vi "ME_acquire_6.vi"() -> ()   [LabVIEW 2015]
doc: "Use this template to build a producer/consumer design pattern. Use this template when you need to execute a process, such as data analysis, when a data source, such as a triggered acquisition, produces data at an uneven rate and you need to execute the process when the data becomes available."
uses:
  Mode.ctl
  oxford_driver/Oxford Drivers/BUSGEN.LLB/OxfordAddress.ctl
  <vilib>/Analysis/baseanly.llb/Mean (DBL).vi
  <vilib>/Utility/file.llb/Write Delimited Spreadsheet (DBL).vi
  <vilib>/express/express arith-compare/Formula/XNode/ExpressFormulaBlockNode.xnode
  <vilib>/gmath/NI_Gmath.lvlib
  <vilib>/Analysis/NI_AALBase.lvlib
panel:
  out "I(B) /Averaged/ 2":cluster{"B array":dbl[], dbl[]}[](graph)
  out "Averaged I(B)":dbl[][](array[numeric])
  out "P(uC/mm^2)":dbl[](array[numeric])
  in  "Sweep Field":bool
  out "P(B)":cluster{"yi":dbl[], dbl[]}(graph)
  out "Offset array":dbl[](array[numeric])
  in  "stop 2":bool
  in  "dB":dbl=0.005
  in  "Dwell Time (ms)":u32=1
  out "appended array":dbl[][](array[numeric])
  in  "Magnet":bool
  out "Actual B Field (T)":dbl
  out "Actual Temperature (K)":dbl
  out "Actual Current (pA)":dbl
  in  "Tab Control":T1(tab)
  out "P(T)":cluster{"yi":dbl[], dbl[]}(graph)
  out "I(T)":cluster{dbl[], dbl[]}(graph)
  in  "Set temperature (K)":dbl=4.5
  in  "Temp Ramping Rate (K/min)":dbl=10.0
  in  "Heater Range":enum16{"Off", "Low", "Medium", "High"}(ring)
  in  "Heater On/Off":bool
  out "I(B) /Averaged/":cluster{"B array":dbl[], dbl[]}[](graph)
  out "I(B) 3":cluster{dbl[], dbl[]}[](graph)
  in  "Go to Set":bool
  in  "Set Field (T)":dbl=0.3
  in  "Field To Zero":bool
  in  "Sweep Rate (T/min)":dbl=2.0 format="%.6f"
  in  "Min Field (T)":dbl
  in  "Max Field (T)":dbl
  out "Up/Down":bool
  in  "Measure Noise":bool
  in  "Cycles":i32
  in  "maximum value":dbl=10.0 format="%0.2f"
  in  "minimum value":dbl=-10.0 format="%0.2f"
  in  "physical channels":tag="Dev1/ai1"
  out "PSD (pA/Hz^1/2) Peaks Removed":cluster{"f0":dbl, "df":dbl, "magnitude":dbl[]}(graph)
  out "PSD (pA/Hz^1/2)":cluster{"f0":dbl, "df":dbl, "magnitude":dbl[]}(graph)
  out "Current (pA) Filtered":waveform(dbl)(graph)
  out "Current (pA)":dbl[](graph)
  in  "Samples per channel":i32=1000
  in  "Rate":dbl=1000.0 format="%0.2f"
  in  "Cut-Off Frequency":dbl=100.0 caption="Lower Cut-Off"
  in  "Filter On":bool
  out "Dc offset":dbl
  in  "Calibrate":bool
  in  "IV converter":refnum<visa-resource-name>="GPIB0::20::INSTR"
  in  "Magnetic Field":refnum<visa-resource-name>="GPIB0::21::INSTR"
  out "Time Lag":dbl=0.0500025749206543
  in  "Lake Shore":refnum<visa-resource-name>="GPIB0::11::INSTR"
  in  "Temp Refresh (s)":dbl=1.0
  in  "Sampling rate (Hz)":dbl=10.0
  in  "Gain (V/A)":dbl=1000000000.0
  in  "Sample area (mm^2)":dbl=3.9
  out "B_V":cluster{dbl[], "Best Linear Fit":dbl[]}[](graph)=[{[-0.00854253601, 0.00626134724, 0.0219834428, 0.0379117736, 0.0535871506, 0.0694316728, 0.0851615152, 0.100816481, 0.116478038, 0.132148461, 0.147876163, 0.16341701, 0.178976744, 0.194563632, 0.210251739, 0.225738944, 0.241298253, 0.256806034, 0.272344374, 0.287933477, 0.303494709, 0.318997125, 0.334591297, 0.350146681, 0.365618053, 0.380940961, 0.39666457, 0.412213675, 0.427724671, 0.443221444, 0.458760641, 0.474360042, 0.489915118, 0.505330598, 0.520967119, 0.536347531, 0.551813711, 0.567441155, 0.582995861, 0.598507522, 0.614041988, 0.629563151, 0.645106262, 0.660611914, 0.676136149, 0.691553948, 0.7071244, 0.72262999, 0.738171137, 0.753700392, 0.76919513, 0.784778028, 0.800215944, 0.8156961, 0.831325434, 0.846852183, 0.862326812, 0.877819169, 0.893312568, 0.90888536, 0.924354789], "Best Linear Fit"=[0.0, 0.005, 0.01, 0.015, 0.02, 0.025, 0.03, 0.035, 0.04, 0.045, 0.05, 0.055, 0.06, 0.065, 0.07, 0.075, 0.08, 0.085, 0.09, 0.095, 0.1, 0.105, 0.11, 0.115, 0.12, 0.125, 0.13, 0.135, 0.14, 0.145, 0.15, 0.155, 0.16, 0.165, 0.17, 0.175, 0.18, 0.185, 0.19, 0.195, 0.2, 0.205, 0.21, 0.215, 0.22, 0.225, 0.23, 0.235, 0.24, 0.245, 0.25, 0.255, 0.26, 0.265, 0.27, 0.275, 0.28, 0.285, 0.29, 0.295, 0.3]}, {[-0.00854253601, 0.00626134724, 0.0219834428, 0.0379117736, 0.0535871506, 0.0694316728, 0.0851615152, 0.100816481, 0.116478038, 0.132148461, 0.147876163, 0.16341701, 0.178976744, 0.194563632, 0.210251739, 0.225738944, 0.241298253, 0.256806034, 0.272344374, 0.287933477, 0.303494709, 0.318997125, 0.334591297, 0.350146681, 0.365618053, 0.380940961, 0.39666457, 0.412213675, 0.427724671, 0.443221444, 0.458760641, 0.474360042, 0.489915118, 0.505330598, 0.520967119, 0.536347531, 0.551813711, 0.567441155, 0.582995861, 0.598507522, 0.614041988, 0.629563151, 0.645106262, 0.660611914, 0.676136149, 0.691553948, 0.7071244, 0.72262999, 0.738171137, 0.753700392, 0.76919513, 0.784778028, 0.800215944, 0.8156961, 0.831325434, 0.846852183, 0.862326812, 0.877819169, 0.893312568, 0.90888536, 0.924354789], "Best Linear Fit"=[-0.00022554388023060128, 0.004536267537808887, 0.009593430775915074, 0.014716931562355689, 0.01975906732634002, 0.024855610270593523, 0.029915265354287977, 0.03495083565949541, 0.03998852608757118, 0.045029068349812316, 0.05008803495326229, 0.055086897848955874, 0.060091835929837946, 0.06510550835596321, 0.07015173884687344, 0.07513334727738563, 0.08013814865293042, 0.08512637555172443, 0.0901244320467579, 0.09513881694893507, 0.10014423687592358, 0.10513073807087174, 0.11014675346564809, 0.1151502923271957, 0.12012680792099008, 0.1250555686413888, 0.1301132186920259, 0.13511473785283767, 0.14010399888730068, 0.14508868495702945, 0.1500870171143548, 0.15510471446726903, 0.16010815425765457, 0.16506669165212906, 0.17009632901003072, 0.1750435864450521, 0.18001843198211442, 0.1850451496356715, 0.19004847041199868, 0.1950379453501071, 0.20003475573578386, 0.20502728708357412, 0.21002687821664084, 0.21501442030211, 0.220007939788244, 0.2249672231113706, 0.22997560874002893, 0.23496313088260184, 0.23996209027618054, 0.24495722449359253, 0.24994125598600042, 0.2549536449902534, 0.25991939913989753, 0.2648987401917687, 0.26992606578200207, 0.2749203939204135, 0.2798979571595809, 0.2848812227804405, 0.2898648235706211, 0.2948739618827834, 0.2998498524919418]}]
  out "V_I":cluster{dbl[], "Best Linear Fit":dbl[]}[](graph)=[{[0.0, 0.035, 0.069, 0.104, 0.138, 0.173, 0.208, 0.242, 0.277, 0.311, 0.346, 0.38, 0.415, 0.45, 0.484, 0.519, 0.553, 0.588, 0.623, 0.657, 0.692, 0.726, 0.761, 0.796, 0.83, 0.865, 0.899, 0.934, 0.969, 1.003, 1.038, 1.072, 1.107, 1.141, 1.176, 1.211, 1.245, 1.28, 1.314, 1.349, 1.384, 1.418, 1.453, 1.487, 1.522, 1.557, 1.591, 1.626, 1.66, 1.695, 1.73, 1.764, 1.799, 1.833, 1.868, 1.902, 1.937, 1.972, 2.006, 2.041, 2.075], "Best Linear Fit"=[-0.00854253601, 0.00626134724, 0.0219834428, 0.0379117736, 0.0535871506, 0.0694316728, 0.0851615152, 0.100816481, 0.116478038, 0.132148461, 0.147876163, 0.16341701, 0.178976744, 0.194563632, 0.210251739, 0.225738944, 0.241298253, 0.256806034, 0.272344374, 0.287933477, 0.303494709, 0.318997125, 0.334591297, 0.350146681, 0.365618053, 0.380940961, 0.39666457, 0.412213675, 0.427724671, 0.443221444, 0.458760641, 0.474360042, 0.489915118, 0.505330598, 0.520967119, 0.536347531, 0.551813711, 0.567441155, 0.582995861, 0.598507522, 0.614041988, 0.629563151, 0.645106262, 0.660611914, 0.676136149, 0.691553948, 0.7071244, 0.72262999, 0.738171137, 0.753700392, 0.76919513, 0.784778028, 0.800215944, 0.8156961, 0.831325434, 0.846852183, 0.862326812, 0.877819169, 0.893312568, 0.90888536, 0.924354789]}, {[0.0, 0.035, 0.069, 0.104, 0.138, 0.173, 0.208, 0.242, 0.277, 0.311, 0.346, 0.38, 0.415, 0.45, 0.484, 0.519, 0.553, 0.588, 0.623, 0.657, 0.692, 0.726, 0.761, 0.796, 0.83, 0.865, 0.899, 0.934, 0.969, 1.003, 1.038, 1.072, 1.107, 1.141, 1.176, 1.211, 1.245, 1.28, 1.314, 1.349, 1.384, 1.418, 1.453, 1.487, 1.522, 1.557, 1.591, 1.626, 1.66, 1.695, 1.73, 1.764, 1.799, 1.833, 1.868, 1.902, 1.937, 1.972, 2.006, 2.041, 2.075], "Best Linear Fit"=[-0.007846580254753975, 0.007882153481927697, 0.02316149482613275, 0.03889022856281441, 0.054169569907019474, 0.06989830364370113, 0.08562703738038281, 0.10090637872458785, 0.11663511246126955, 0.1319144538054746, 0.14764318754215625, 0.1629225288863613, 0.17865126262304296, 0.19437999635972467, 0.2096593377039297, 0.22538807144061138, 0.24066741278481643, 0.25639614652149806, 0.27212488025817977, 0.2874042216023848, 0.3031329553390665, 0.31841229668327153, 0.3341410304199532, 0.3498697641566349, 0.3651491055008399, 0.3808778392375216, 0.39615718058172666, 0.4118859143184083, 0.42761464805509, 0.442893989399295, 0.45862272313597674, 0.4739020644801818, 0.48963079821686345, 0.5049101395610684, 0.5206388732977502, 0.5363676070344319, 0.5516469483786369, 0.5673756821153185, 0.5826550234595236, 0.5983837571962053, 0.6141124909328869, 0.629391832277092, 0.6451205660137737, 0.6603999073579787, 0.6761286410946604, 0.691857374831342, 0.7071367161755471, 0.7228654499122288, 0.7381447912564338, 0.7538735249931156, 0.7696022587297972, 0.7848816000740022, 0.8006103338106839, 0.815889675154889, 0.8316184088915707, 0.8468977502357756, 0.8626264839724573, 0.878355217709139, 0.893634559053344, 0.9093632927900257, 0.9246426341342309]}]
  out "B0 (T)":dbl=0.0025222449819540214
  out "B/V (T/V)":dbl=0.321659617116981
  out "I0 (A)":dbl=-0.007846580254753975
  out "V/I (Ohm)":dbl=0.44939239247661916
  in  "Offset?":bool
  in  "Temp/Magnetic Field":bool
  out "Save":dbl[][](array[numeric])
  out "output array":dbl[][](array[numeric])
  out "index":i8
  out "Read?":bool
  out "Magnetic Field (T)":dbl[](array[numeric])
  out "Reset":bool
  out "Measured Current (pA)":dbl[](array[numeric])
  out "Elapsed Time (s)":dbl[](array[numeric])
  out "Start time":timestamp
  in  "Enum":T2=enum."Process"
  out "B array":dbl[](array[numeric])
  in  "dB (T)":dbl=0.0001
  in  "Counter":i8
  out "L magnet (H)":dbl
  out "R magnet (mOhm)":dbl
  out "Actual Current (R0)":dbl
  out "Actual Field (T)":dbl
  out "Temperature array":dbl[](array[numeric])
  in  "New Measurement File":bool
  out "Measurement File":path
  out "refnum out":refnum<file>
  in  "Measuring":bool
  in  "Measure (Start/Pause)":bool
  in  "stop":bool
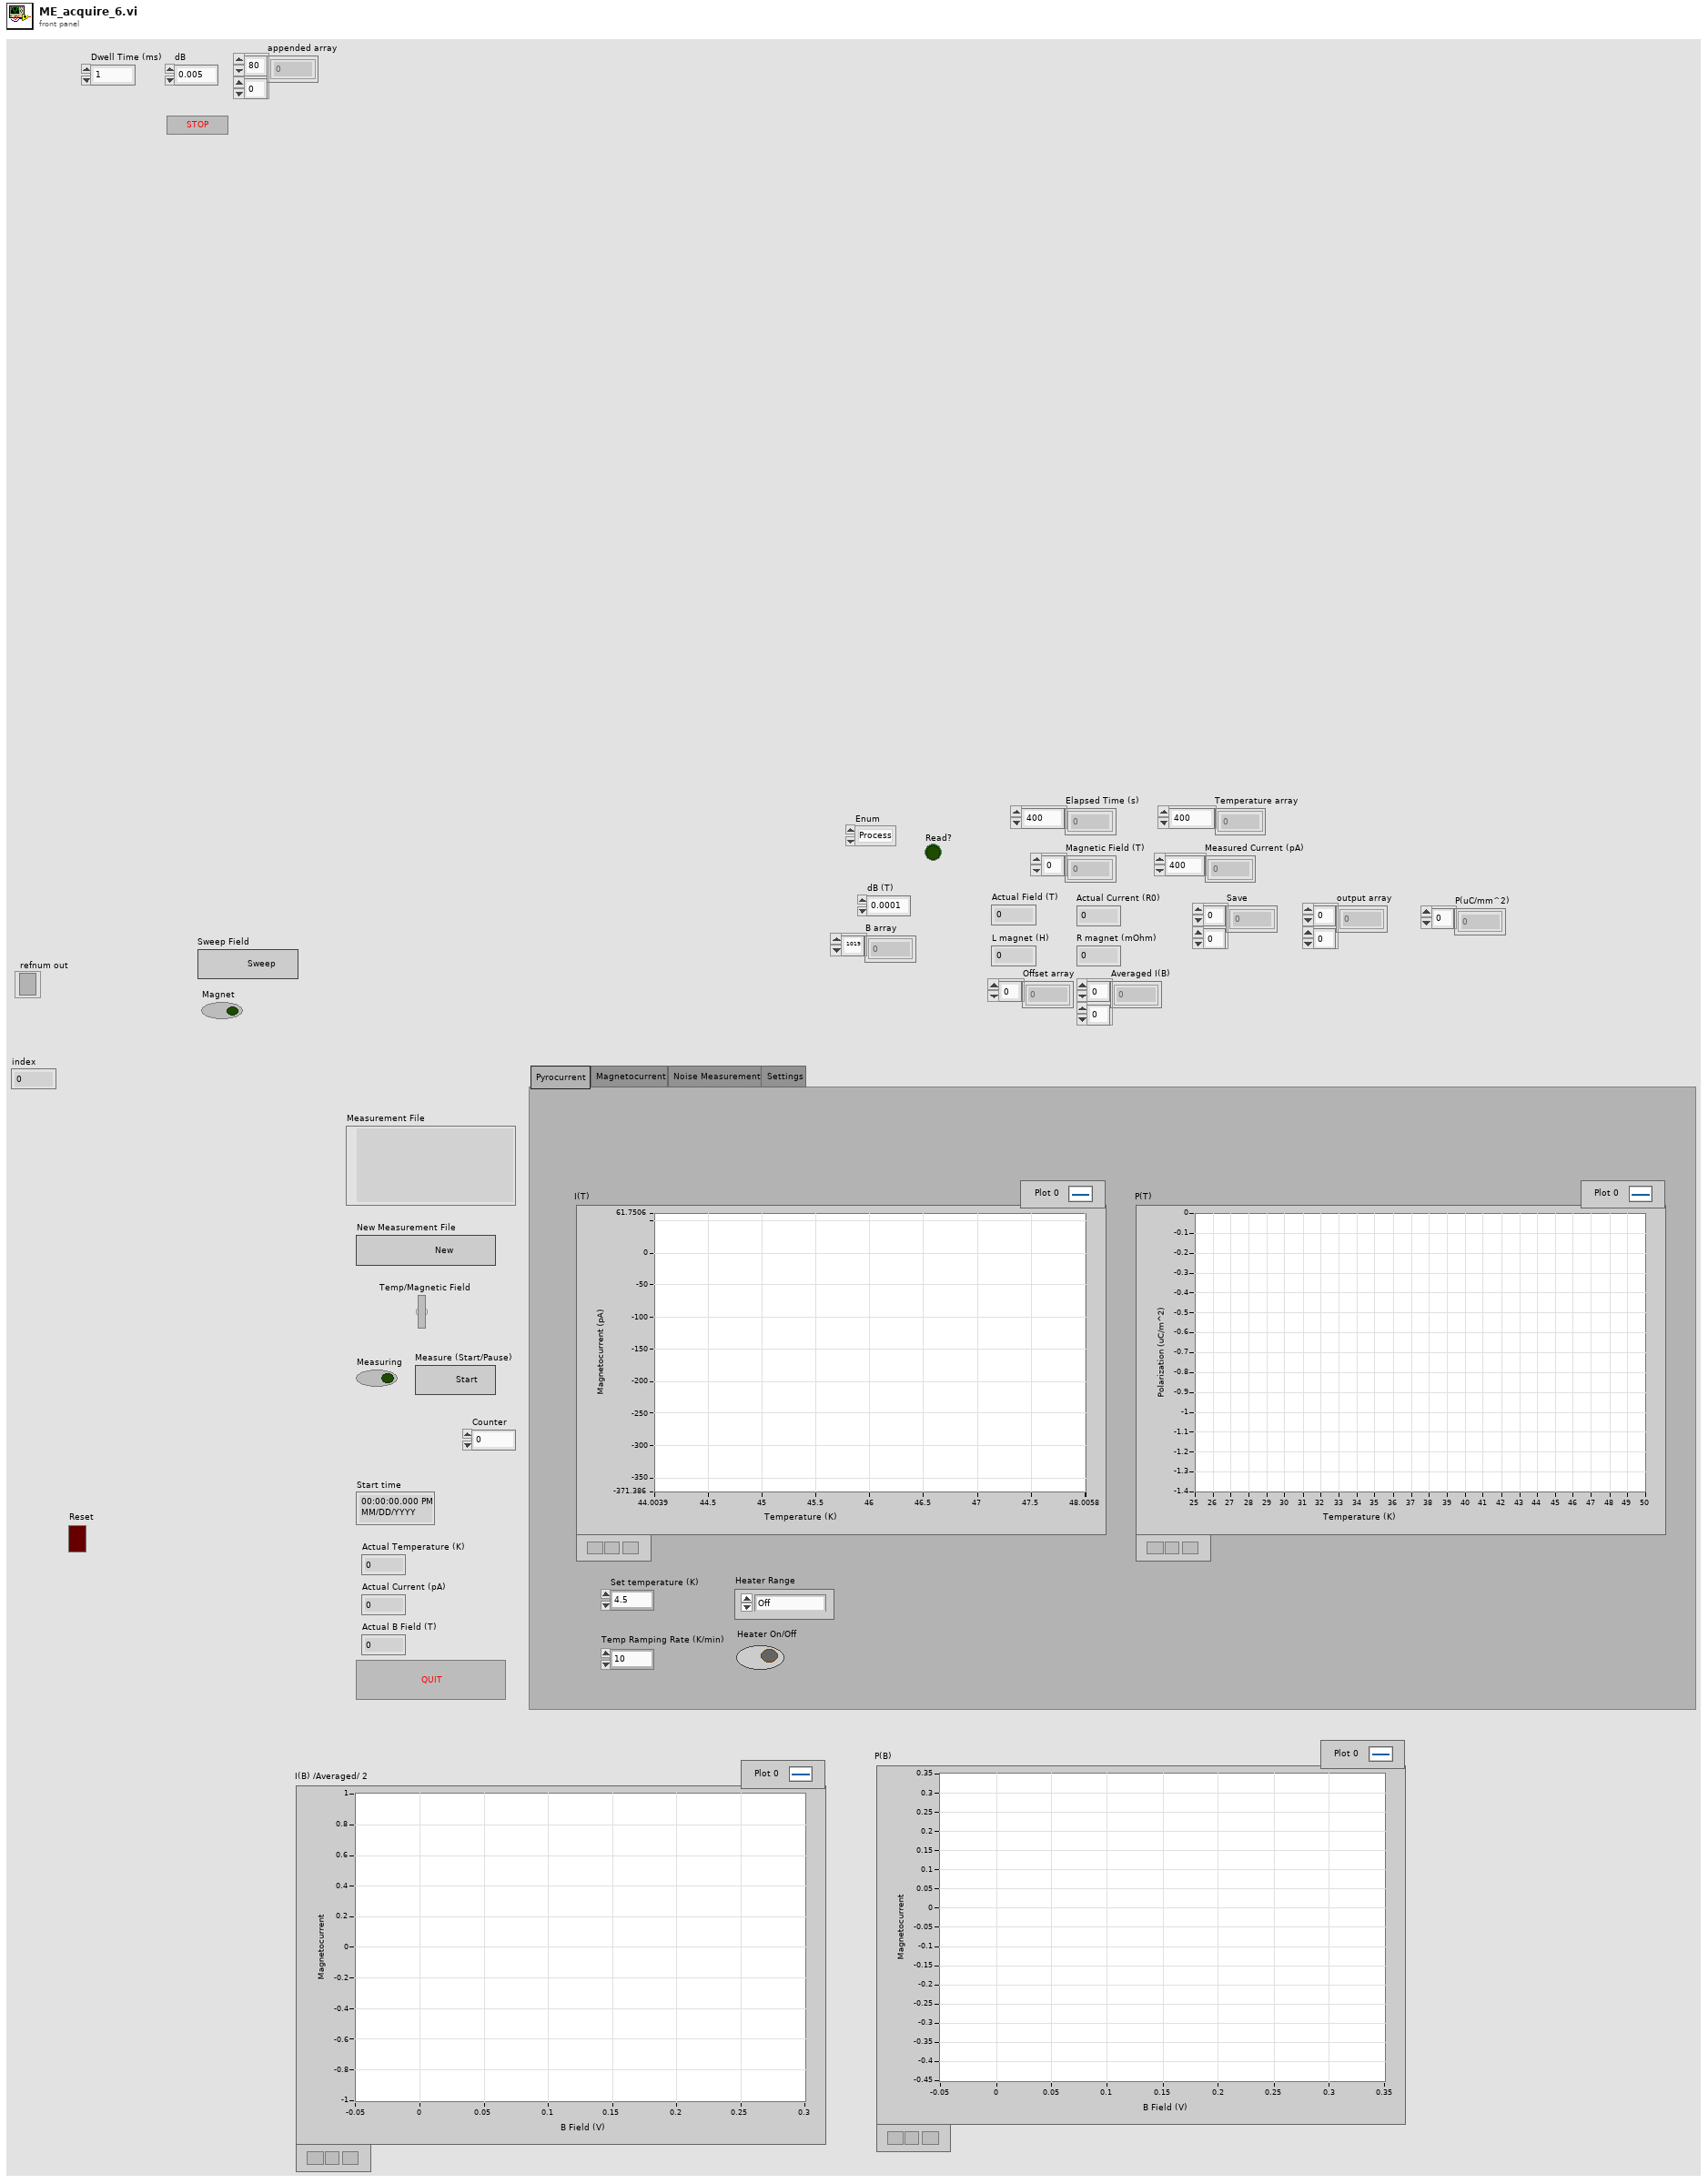
[diagram p1: front panel]
types:
  T1 = enum32{"Pyrocurrent", "Magnetocurrent", "Noise Measurement", "Settings"}
  T2 = typedef "Mode.ctl" = enum16{"Offset", "Process", "Sweep", "Plot", "Save", "Return"}
  T3 = enum16{"open", "replace", "create", "open or create", "replace or create", "replace or create with confirmation"}
  T4 = typedef "OxfordAddress.ctl" = cluster{"Com Port":i32, "ISOBUS Address":i32, "GPIB Address":i16, "Communication":enum16{"RS232", "ISOBUS", "GPIB", "Gateway"}}
  T5 = cluster{"seconds since 1Jan1904":timestamp, "read buffer":string, "read buffer":string}
  T6 = cluster{"B array":dbl[], "Averaged I(B) out":dbl[]}
  T7 = cluster{"B array":dbl[], "Averaged I(B) out":dbl[]}[]
  T8 = cluster{"I array out (A)":dbl[], "V array out (V)":dbl[]}
  T9 = cluster{"I array out (A)":dbl[], "Best Linear Fit":dbl[]}
  T10 = cluster{"V array out (V)":dbl[], "B array Out":dbl[]}
  T11 = cluster{"V array out (V)":dbl[], "Best Linear Fit 2":dbl[]}
  T12 = cluster{"I array out (A)":dbl[], "Best Linear Fit":dbl[]}[]
  T13 = cluster{"V array out (V)":dbl[], "Best Linear Fit 2":dbl[]}[]
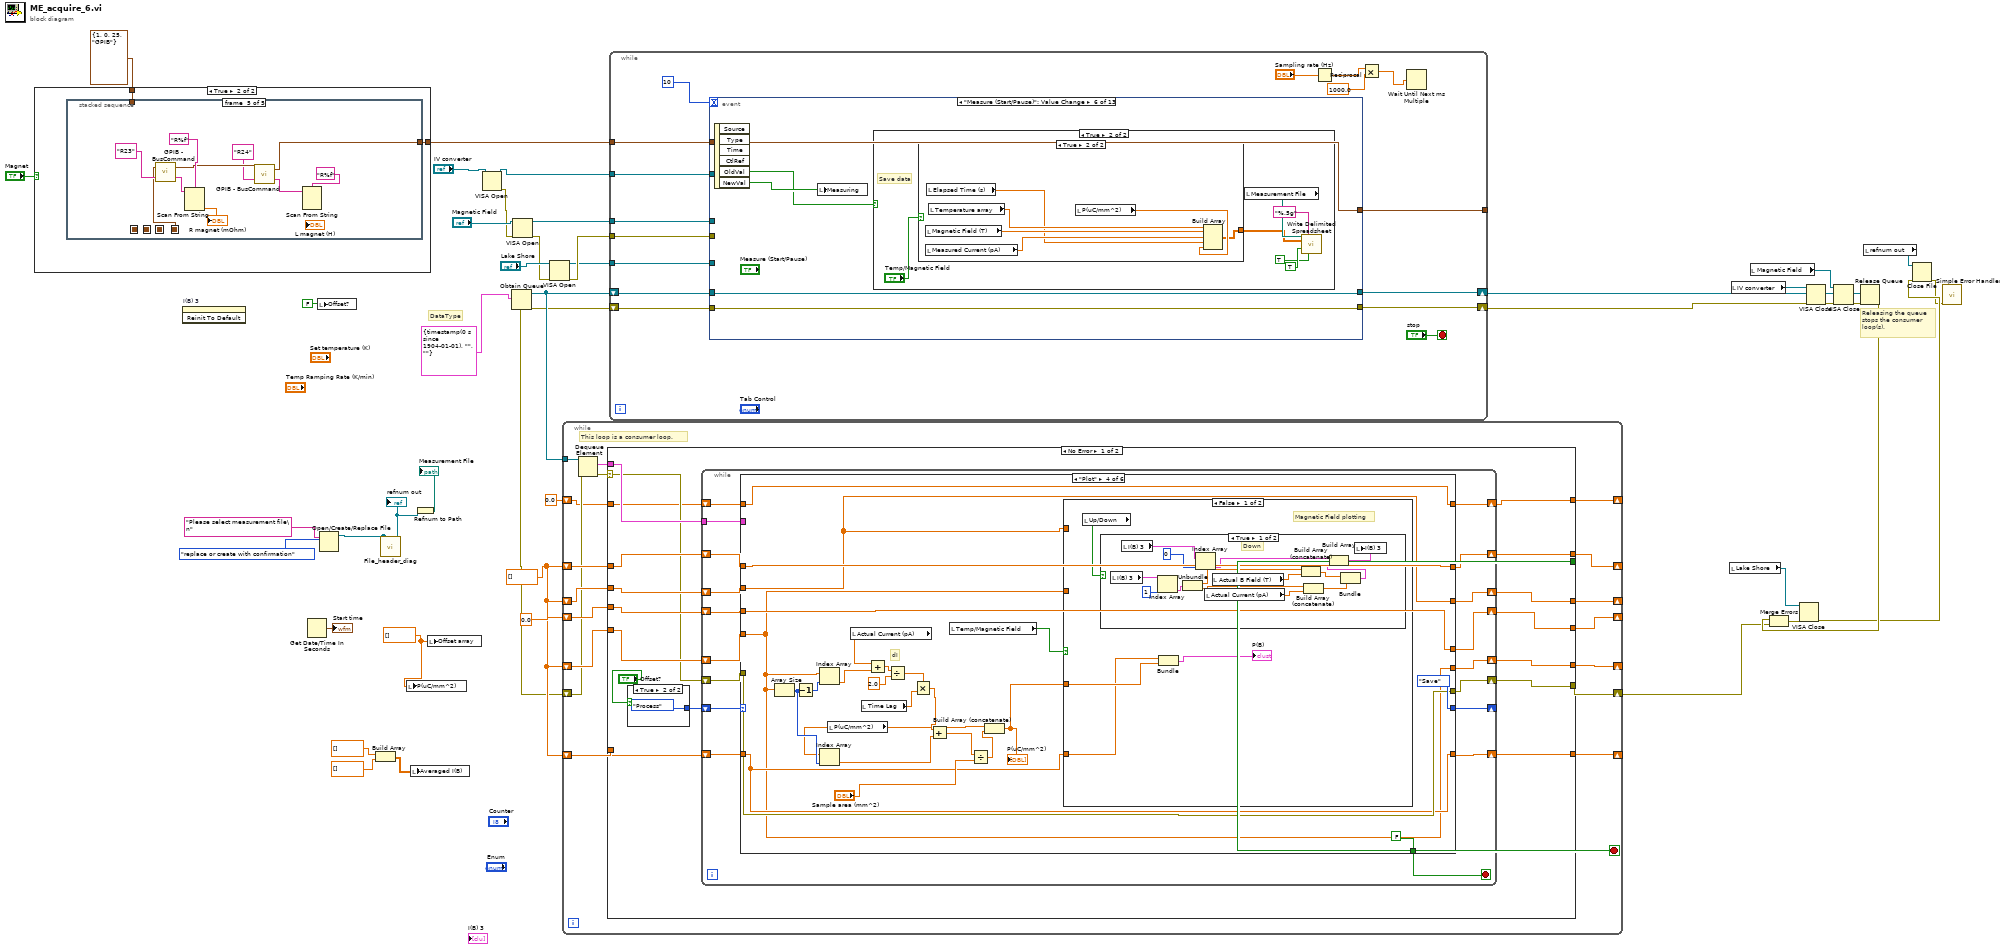
[diagram p0: block diagram]
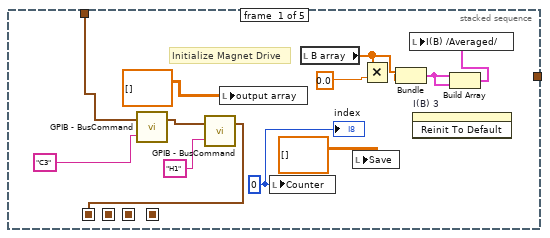
[diagram p3: hidden frame]
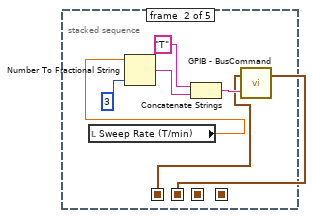
[diagram p4: hidden frame]
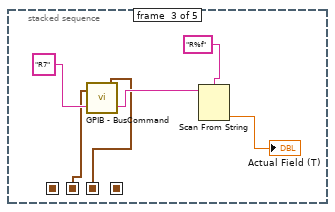
[diagram p5: hidden frame]
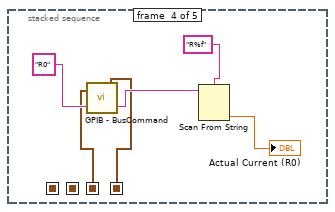
[diagram p6: hidden frame]
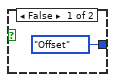
[diagram p7: hidden frame]
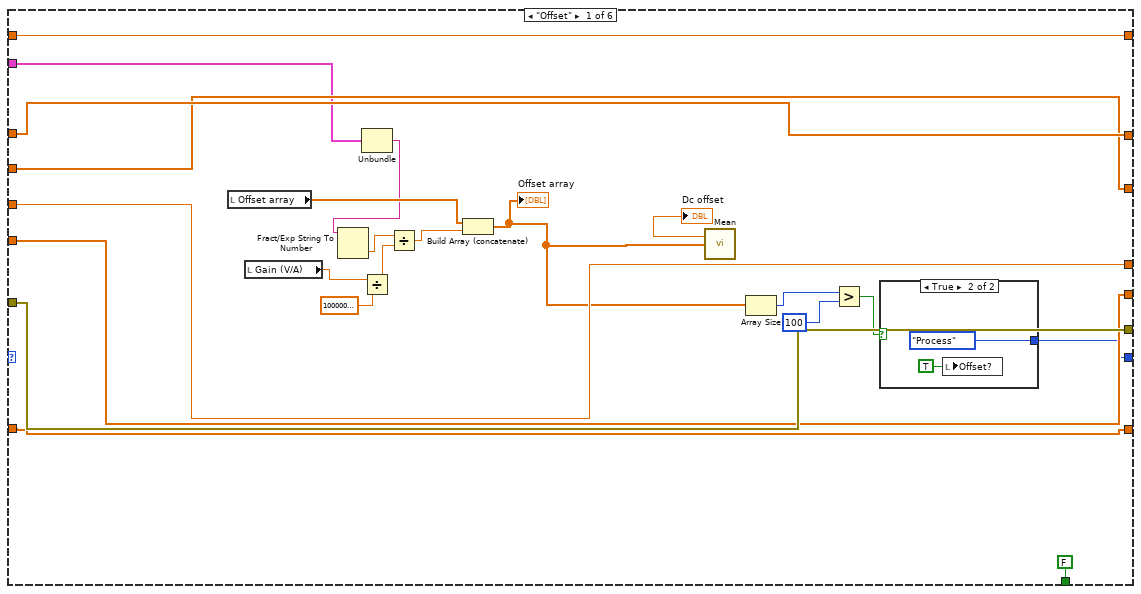
[diagram p8: hidden frame]
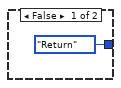
[diagram p9: hidden frame]
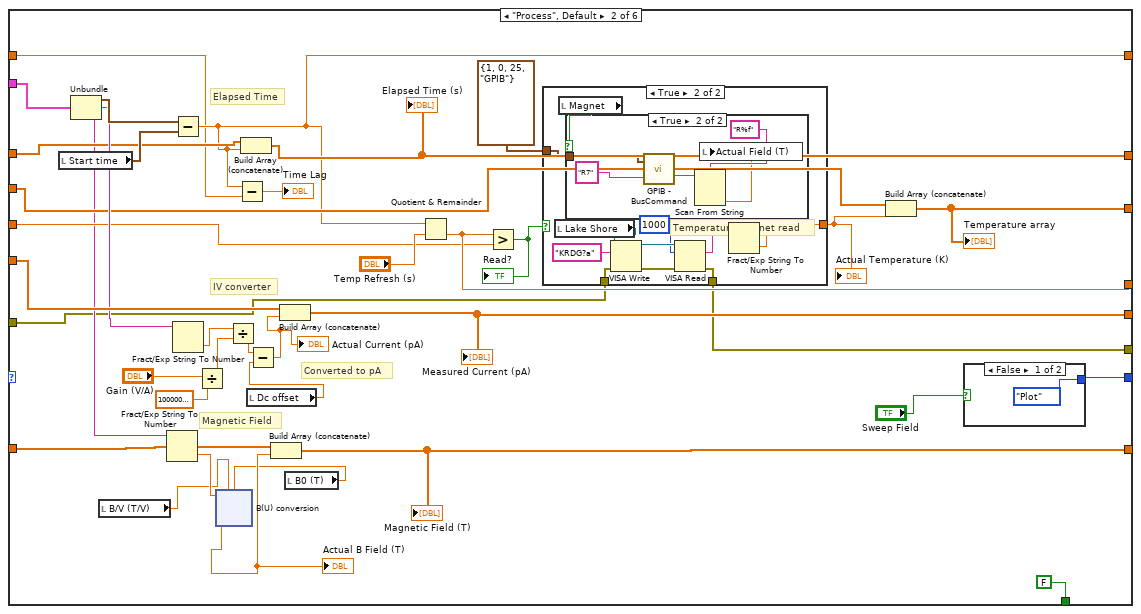
[diagram p10: hidden frame]
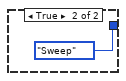
[diagram p11: hidden frame]
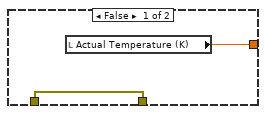
[diagram p12: hidden frame]
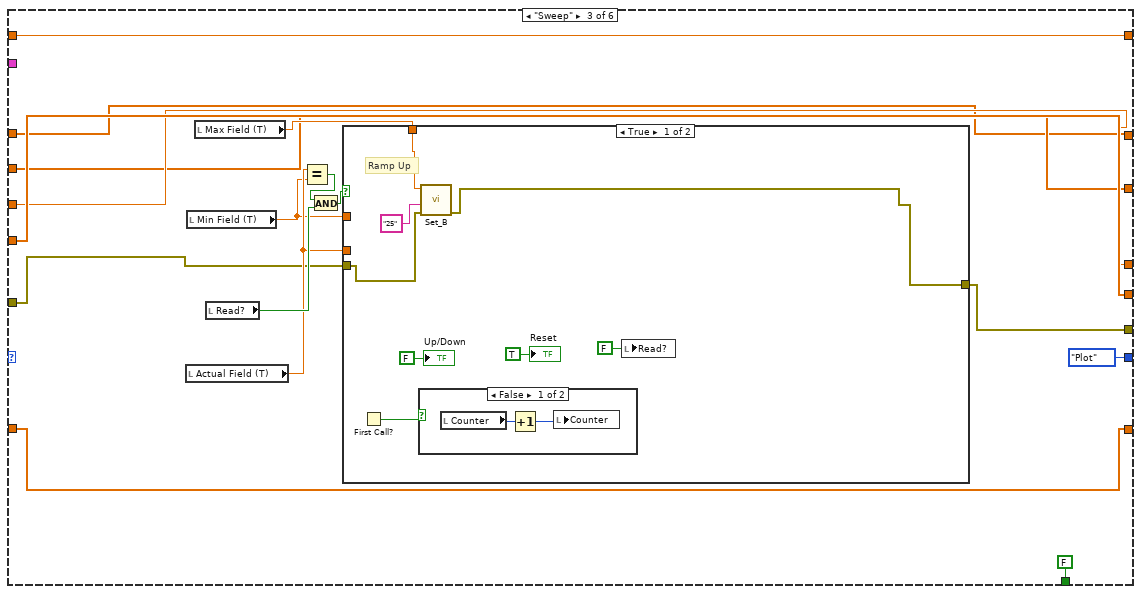
[diagram p14: hidden frame]
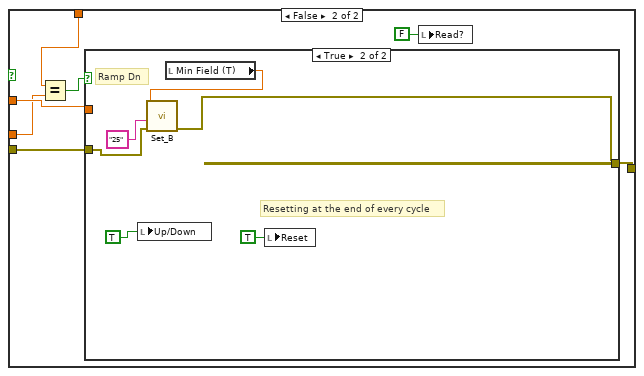
[diagram p16: hidden frame]
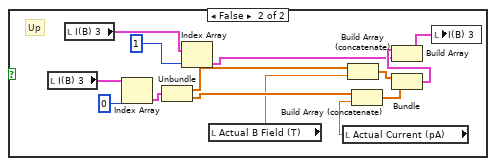
[diagram p18: hidden frame]
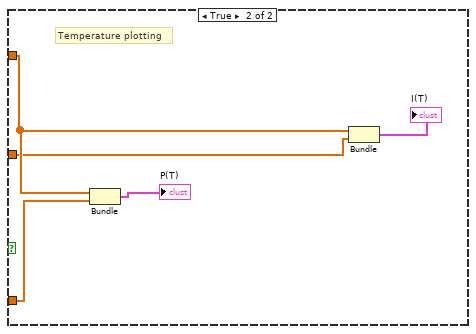
[diagram p19: hidden frame]
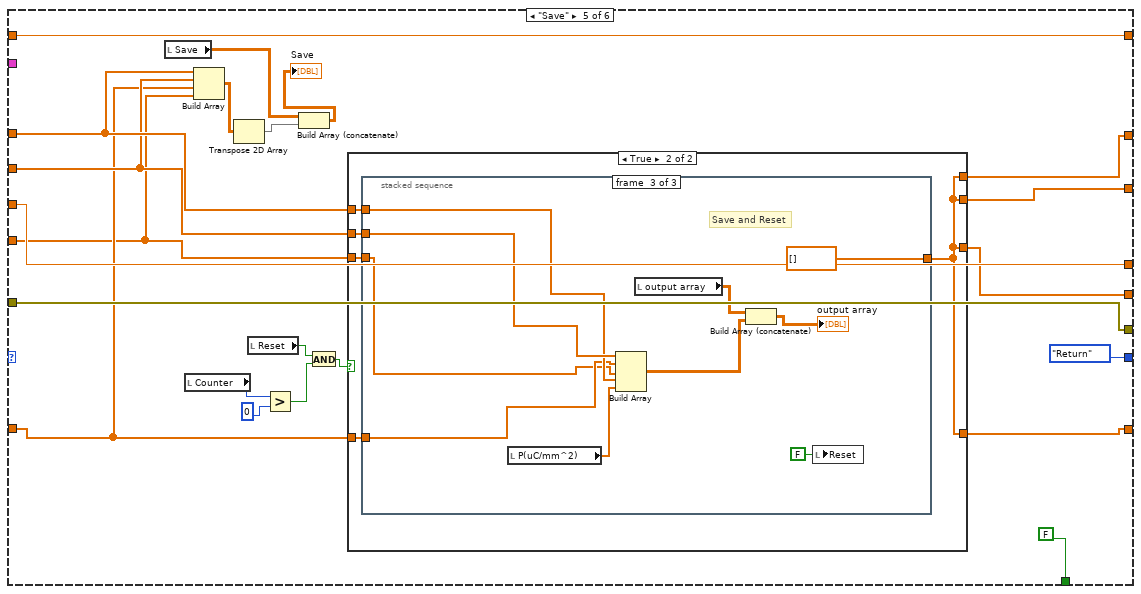
[diagram p20: hidden frame]
diagram:
  w4 = dbl[] []
  w11 = dbl[] []
  # "DataType"
  # "Releasing the queue stops the consumer loop(s)."
  n1 = case shown="True" "Magnet" {
    tunnel: T4 {"Com Port"=1, "ISOBUS Address"=0, "GPIB Address"=25, "Communication"=enum."GPIB"} ("Address") -> [w42 w44]
    tunnel: [w42 w43] -> w20
    frame False {
    }
    frame True {
      n2 = stacked-sequence {
        seq-local: [w54 _ _ _ _] -> [_ w59 _ _ _]
        seq-local: [_ w58 _ _ _] -> [_ _ w66 _ _]
        seq-local: [_ _ w65 _ _] -> [_ _ _ w72 _]
        seq-local: [_ _ _ w71 _] -> [_ _ _ _ w82]
        tunnel: w44 -> [w56 _ _ _ _]
        tunnel: [_ _ _ _ w80] -> w43
        frame #0 {
          w52 = i8 0 ("Counter")
          # "Initialize Magnet Drive"
          n3 = call "GPIB - BusCommand.vi"("Command"="C3", "Address"=w56) -> ("Address(thru)"=w55:T4)  [unwired: 1 out]
          n4 = call "GPIB - BusCommand.vi"("Command"="H1", "Address"=w55) -> ("Address(thru)"=w54:T4)  [unwired: 1 out]
          n5 = local write "output array"(dbl[][] []) -> ()
          n6 = local write "Counter"(w52) -> ()
          n7 = local read "B array"() -> (w50:dbl[])
          n8 = local write "Save"(dbl[][] [] ("Save")) -> ()
          n9 = Multiply(x=w50, y=0.0) -> (x*y=w49:dbl[])
          n10 = Bundle("B array"=w50, w49) -> (w48:cluster{"B array":dbl[], dbl[]})  [unwired: 1 in]
          n11 = invoke on="I(B) 3" class="XYGraph (strict)" method="Reinit To Default"() -> ()  [unwired: 3 in, 3 out]
          n12 = Build Array(w48, w48) -> (w47:cluster{"B array":dbl[], dbl[]}[])
          n13 = local write "I(B) /Averaged/"(w47) -> ()
          "index" <- w52
        }
        frame #1 {
          n14 = local read "Sweep Rate (T/min)"() -> (w60:dbl)
          n15 = Number To Fractional String(number=w60, precision (6)=i16 3) -> (F-format string=w62:string)  [unwired: 2 in]
          n16 = Concatenate Strings("T" ("format string"), w62) -> (w61:string)
          n17 = call "GPIB - BusCommand.vi"("Command"=w61, "Address"=w59) -> ("Address(thru)"=w58:T4)  [unwired: 1 out]
        }
        frame #2 {
          n18 = call "GPIB - BusCommand.vi"("Command"="R7" ("format string"), "Address"=w66) -> ("Reply"=w70:string, "Address(thru)"=w65:T4)
          n19 = Scan From String(format string="R%f" ("remaining string"), input string=w70) -> (output 1=→"Actual Field (T)":dbl)  [unwired: 3 in, 3 out]
        }
        frame #3 {
          n20 = call "GPIB - BusCommand.vi"("Command"="R0" ("format string"), "Address"=w72) -> ("Reply"=w76:string, "Address(thru)"=w71:T4)
          n21 = Scan From String(format string="R%f" ("remaining string"), input string=w76) -> (output 1=→"Actual Current (R0)":dbl)  [unwired: 3 in, 3 out]
        }
        frame #4 {
          n22 = call "GPIB - BusCommand.vi"("Command"="R23" ("format string"), "Address"=w82) -> ("Reply"=w86:string, "Address(thru)"=w81:T4)
          n23 = Scan From String(format string="R%f" ("remaining string"), input string=w86) -> (output 1=→"R magnet (mOhm)":dbl)  [unwired: 3 in, 3 out]
          n24 = call "GPIB - BusCommand.vi"("Command"="R24" ("format string"), "Address"=w81) -> ("Reply"=w78:string, "Address(thru)"=w80:T4)
          n25 = Scan From String(format string="R%f" ("remaining string"), input string=w78) -> ()  [unwired: 4 in, 3 out]
        }
      }
    }
  }
  n26 = invoke on="I(B) 3" class="XYGraph (strict)" method="Reinit To Default"() -> ()  [unwired: 3 in, 3 out]
  n27 = Get Date/Time In Seconds() -> (seconds since 1Jan1904=→"Start time":timestamp)
  n28 = local write "Offset?"(FALSE ("Offset?")) -> ()
  n29 = Open/Create/Replace File(prompt="Please select measurement file\n", operation (0:open)=T3."replace or create with confirmation") -> (refnum out=w16:refnum<file>)  [unwired: 4 in, 2 out]
  "refnum out" <- w16
  n30 = Build Array(dbl[] [], dbl[] []) -> (w1:dbl[][])
  n31 = call "File_header_diag.vi"("Byte Stream File in"=w16) -> ()  [unwired: 11 in]
  n32 = local write "P(uC/mm^2)"(w4) -> ()
  n33 = local write "Averaged I(B)"(w1) -> ()
  n34 = Refnum to Path(1:w16) -> (0:→"Measurement File":path)
  n35 = local write "Offset array"(w4) -> ()
  n36 = VISA Open(VISA resource name="IV converter") -> (VISA resource name=w36:refnum<visa-resource-name>, error out=w38:errorcluster)  [unwired: 4 in]
  n37 = Obtain Queue(element data type=T5 {"seconds since 1Jan1904"=timestamp(0 s since 1904-01-01), "read buffer"="", "read buffer"=""} ("output cluster")) -> (queue out=w41:refnum<queue>, error out=w9:errorcluster)  [unwired: 4 in, 1 out]
  n38 = VISA Open(error in (no error)=w38, VISA resource name="Magnetic Field") -> (VISA resource name=w35:refnum<visa-resource-name>, error out=w13:errorcluster)  [unwired: 3 in]
  n39 = VISA Open(error in (no error)=w13, VISA resource name="Lake Shore") -> (VISA resource name=w7:refnum<visa-resource-name>, error out=w12:errorcluster)  [unwired: 3 in]
  n40 = while {
    tunnel: w41 -> [w104]
    shift-right: [w99] -> _
    shift-left: w11 -> [w98]
    shift-right: [w97] -> _
    shift-left: w11 -> [w96]
    shift-right: [w95] -> _
    shift-left: w11 -> [w94]
    shift-right: [w93] -> _
    shift-left: 0.0 -> [w92]
    shift-right: [w91] -> _
    shift-left: w11 -> [w90]
    shift-right: [w100] -> w25
    shift-left: w9 -> [w89]
    shift-right: [w88] -> _
    shift-left: 0.0 -> [w87]
    stop <- w101 stop-if-true
    # "This loop is a consumer loop."
    n41 = Dequeue Element(queue=w104, error in (no error)=w89) -> (element=w102:T5, error out=w103:errorcluster)  [unwired: 1 in, 2 out]
    n42 = case shown="No Error" w103 {
      selector: w103 -> [w109 w443]
      tunnel: w102 -> [w120 _]
      tunnel: [_ TRUE] -> w101
      tunnel: [w108 w443] -> w100
      tunnel: [w119 w442] -> w99
      tunnel: w98 -> [w118 w442]
      tunnel: [w117 w439] -> w97
      tunnel: w96 -> [w116 w439]
      tunnel: [w115 w438] -> w95
      tunnel: w94 -> [w114 w438]
      tunnel: [w113 w440] -> w93
      tunnel: w92 -> [w112 w440]
      tunnel: [w111 w441] -> w91
      tunnel: w90 -> [w110 w441]
      tunnel: [w107 w437] -> w88
      tunnel: w87 -> [w106 w437]
      frame No Error {
        n43 = case shown="True" "Offset?" {
          tunnel: [Mode."Offset" ("Enum") Mode."Process" ("Enum")] -> w121
          frame False {
          }
          frame True {
          }
        }
        n44 = while {
          shift-right: [w129] -> _
          shift-left: w121 -> [w141]
          tunnel: w120 -> [w140]
          shift-right: [w139] -> w119
          shift-left: w118 -> [w138]
          shift-right: [w131] -> w111
          shift-left: w110 -> [w130]
          shift-right: [w133] -> w113
          shift-left: w112 -> [w132]
          shift-right: [w137] -> w117
          shift-left: w116 -> [w136]
          shift-right: [w127] -> w108
          shift-left: w109 -> [w128]
          shift-right: [w135] -> w115
          shift-left: w114 -> [w134]
          shift-right: [w125] -> w107
          shift-left: w106 -> [w124]
          stop <- w126 stop-if-true
          n45 = case shown="\"Plot\"" w141 {
            tunnel: w140 -> [w156 w202 _ _ _ _]
            tunnel: [w163 w199 w239 w301 w347 w435] -> w139
            tunnel: w138 -> [w163 w190 w239 w301 w346 w435]
            tunnel: [w157 w198 w242 w277 w349 w432] -> w137
            tunnel: w136 -> [w157 w197 w242 w277 w343 w432]
            tunnel: [w159 w194 w244 w278 w350 w429] -> w135
            tunnel: w134 -> [w159 w193 w244 w278 w344 w429]
            tunnel: [w161 w189 w241 w300 w358 w433] -> w133
            tunnel: w132 -> [w161 w188 w241 w300 w358 w433]
            tunnel: [w162 w185 w240 w279 w348 w434] -> w131
            tunnel: w130 -> [w162 w186 w240 w279 w345 w434]
            tunnel: [w144 w183 Mode."Plot" ("Enum") Mode."Save" ("Enum") Mode."Return" ("Enum") Mode."Process" ("Enum")] -> w129
            tunnel: w128 -> [w160 w181 w246 w296 w357 w431]
            tunnel: [w160 w180 w245 w296 w357 w431] -> w127
            tunnel: [FALSE FALSE FALSE FALSE FALSE TRUE] -> w126
            tunnel: [w143 w177 w238 w297 w356 w428] -> w125
            tunnel: w124 -> [w143 w176 w238 w297 w356 w428]
            frame "Offset" {
              n46 = local read "Offset array"() -> (w150:dbl[])
              n47 = local read "Gain (V/A)"() -> (w154:dbl)
              n48 = Unbundle(w156) -> ("read buffer"=w142:string)  [unwired: 2 out]
              n49 = Fract/Exp String To Number(string=w142) -> (number=w155:dbl)  [unwired: 3 in, 1 out]
              n50 = Divide(x=w154, y=1000000000000.0) -> (x/y=w152:dbl)
              n51 = Divide(x=w155, y=w152) -> (x/y=w151:dbl)
              n52 = Build Array (concatenate)(w150, w151) -> (w145:dbl[])
              "Offset array" <- w145
              n53 = call-poly <vilib>:"Mean.vi"("X"=w145) -> ("mean"=→"Dc offset":dbl)  [unwired: 1 out]
              n54 = Array Size(array=w145) -> (size(s)=w149:i32)
              n55 = Greater?(x=w149, y=100) -> (0:w147:bool)
              n56 = case shown="True" w147 {
                tunnel: [Mode."Return" ("Enum") Mode."Process" ("Enum")] -> w144
                frame False {
                }
                frame True {
                  n57 = local write "Offset?"(TRUE ("Offset?")) -> ()
                }
              }
            }
            frame "Process", Default {
              # "Converted to pA"
              # "Magnetic Field"
              # "IV converter"
              # "Elapsed Time"
              n58 = local read "Start time"() -> (w200:timestamp)
              n59 = Unbundle(w202) -> ("seconds since 1Jan1904"=w201:timestamp, "read buffer"=w195:string, "read buffer"=w182:string)
              n60 = local read "B/V (T/V)"() -> (w172:dbl)
              n61 = Fract/Exp String To Number(string=w182) -> (number=w192:dbl)  [unwired: 3 in, 1 out]
              n62 = Subtract(x=w201, y=w200) -> (x-y=w177:dbl)
              n63 = Fract/Exp String To Number(string=w195) -> (number=w196:dbl)  [unwired: 3 in, 1 out]
              n64 = Divide(x="Gain (V/A)", y=1000000000000.0) -> (x/y=w175:dbl)
              n65 = Divide(x=w196, y=w175) -> (x/y=w170:dbl)
              n66 = Subtract(x=w177, y=w176) -> (x-y=→"Time Lag":dbl)
              n67 = Build Array (concatenate)(w190, w177) -> (w199:dbl[])
              "Elapsed Time (s)" <- w199
              n68 = local read "Dc offset"() -> (w168:dbl)
              n69 = Subtract(x=w170, y=w168) -> (x-y=w169:dbl)
              "Actual Current (pA)" <- w169
              n70 = Build Array (concatenate)(w197, w169) -> (w198:dbl[])
              "Measured Current (pA)" <- w198
              n71 = local read "B0 (T)"() -> (w171:dbl)
              n72 = xnode "B(U) conversion"("V"=w192, "BpV"=w172, "B0"=w171) -> ("Result"=w191:dbl)  [unwired: 1 in, 1 out]
              "Actual B Field (T)" <- w191
              n73 = Build Array (concatenate)(w193, w191) -> (w194:dbl[])
              "Magnetic Field (T)" <- w194
              n74 = Quotient & Remainder(x=w177, y="Temp Refresh (s)") -> (floor(x/y)=w189:dbl)  [unwired: 1 out]
              n75 = Greater?(x=w189, y=w188) -> (0:w187:bool)
              "Read?" <- w187
              n76 = case shown="True" w187 {
                tunnel: [w208 w214] -> w184
                tunnel: w181 -> [w207 w213]
                tunnel: [w207 w212] -> w180
                tunnel: T4 {"Com Port"=1, "ISOBUS Address"=0, "GPIB Address"=25, "Communication"=enum."GPIB"} ("Address") -> [_ w211]
                frame False {
                  n77 = local read "Actual Temperature (K)"() -> (w208:dbl)
                }
                frame True {
                  # "Temperature/Magnet read"
                  n78 = local read "Lake Shore"() -> (w210:refnum<visa-resource-name>)
                  n79 = local read "Magnet"() -> (w209:bool)
                  n80 = case shown="True" w209 {
                    tunnel: w211 -> [_ w221]
                    frame False {
                    }
                    frame True {
                      n81 = call "GPIB - BusCommand.vi"("Command"="R7" ("format string"), "Address"=w221) -> ("Reply"=w222:string)  [unwired: 1 out]
                      n82 = Scan From String(format string="R%f" ("remaining string"), input string=w222) -> (output 1=w220:dbl)  [unwired: 3 in, 3 out]
                      n83 = local write "Actual Field (T)"(w220) -> ()
                    }
                  }
                  n84 = VISA Write(VISA resource name=w210, write buffer="KRDG?a", error in (no error)=w213) -> (VISA resource name out=w218:refnum<visa-resource-name>, error out=w217:errorcluster)  [unwired: 1 out]
                  n85 = VISA Read(VISA resource name=w218, byte count=u32 1000, error in (no error)=w217) -> (read buffer=w215:string, error out=w212:errorcluster)  [unwired: 2 out]
                  n86 = Fract/Exp String To Number(string=w215) -> (number=w214:dbl)  [unwired: 3 in, 1 out]
                }
              }
              "Actual Temperature (K)" <- w184
              n87 = Build Array (concatenate)(w186, w184) -> (w185:dbl[])
              "Temperature array" <- w185
              n88 = case shown="False" "Sweep Field" {
                tunnel: [Mode."Plot" ("Enum") Mode."Sweep" ("Enum")] -> w183
                frame False {
                }
                frame True {
                }
              }
            }
            frame "Sweep" {
              n89 = local read "Actual Field (T)"() -> (w249:dbl)
              n90 = local read "Min Field (T)"() -> (w248:dbl)
              n91 = local read "Max Field (T)"() -> (w247:dbl)
              n92 = local read "Read?"() -> (w252:bool)
              n93 = Equal?(x=w249, y=w248) -> (x = y?=w250:bool)
              n94 = And(x=w250, y=w252) -> (x .and. y?=w251:bool)
              n95 = case shown="True" w251 {
                tunnel: [w259 w269] -> w245
                tunnel: w247 -> [w260 w268]
                tunnel: w248 -> [_ w267]
                tunnel: w249 -> [_ w265]
                tunnel: w246 -> [w258 w264]
                frame True {
                  # "Ramp Up"
                  n96 = First Call?() -> (First Call?: T/F=w253:bool)
                  n97 = case shown="False" w253 {
                    frame False {
                      n98 = local read "Counter"() -> (w261:i8)
                      n99 = Increment(x=w261) -> (x+1=w262:i8)
                      n100 = local write "Counter"(w262) -> ()
                    }
                    frame True {
                    }
                  }
                  n101 = call "Set_B.vi"("error in (no error)"=w258, "address string"="25", "Set Field (T)"=w260) -> ("error out"=w259:errorcluster)  [unwired: 8 in]
                  n102 = local write "Read?"(FALSE ("Read?")) -> ()
                  "Up/Down" <- FALSE ("Up/Down")
                  "Reset" <- TRUE ("Save")
                }
                frame False {
                  n103 = Equal?(x=w268, y=w265) -> (x = y?=w266:bool)
                  n104 = case shown="True" w266 {
                    tunnel: [w270 w273] -> w269
                    tunnel: w267 -> [_ _]
                    tunnel: w264 -> [w270 w274]
                    frame False {
                    }
                    frame True {
                      # "Resetting at the end of every cycle"
                      # "Ramp Dn"
                      n105 = local write "Up/Down"(TRUE ("Up/Down")) -> ()
                      n106 = local read "Min Field (T)"() -> (w272:dbl)
                      n107 = call "Set_B.vi"("error in (no error)"=w274, "address string"="25", "Set Field (T)"=w272) -> ("error out"=w273:errorcluster)  [unwired: 8 in]
                      n108 = local write "Reset"(TRUE ("Reset")) -> ()
                    }
                  }
                  n109 = local write "Read?"(FALSE ("Read?")) -> ()
                }
              }
            }
            frame "Plot" {
              # "dI"
              n110 = Array Size(array=w277) -> (size(s)=w287:i32)
              n111 = Decrement(x=w287) -> (x-1=w294:i32)
              n112 = Index Array(array=w277, index=w294) -> (element=w292:dbl)
              n113 = local read "P(uC/mm^2)"() -> (w284:dbl[])
              n114 = Index Array(array=w284, index=w287) -> (element=w285:dbl)
              n115 = local read "Actual Current (pA)"() -> (w293:dbl)
              n116 = local read "Time Lag"() -> (w288:dbl)
              n117 = Add(x=w293, y=w292) -> (x+y=w291:dbl)
              n118 = Divide(x=w291, y=2.0) -> (x/y=w289:dbl)
              n119 = Multiply(x=w289, y=w288) -> (x*y=w286:dbl)
              n120 = Add(x=w286, y=w285) -> (x+y=w283:dbl)
              n121 = local read "Temp/Magnetic Field"() -> (w295:bool)
              n122 = Divide(x=w283, y="Sample area (mm^2)") -> (x/y=w282:dbl)
              n123 = Build Array (concatenate)(w284, w282) -> (w280:dbl[])
              "P(uC/mm^2)" <- w280
              n124 = case shown="False" w295 {
                tunnel: w279 -> [_ w336]
                tunnel: w278 -> [w302 _]
                tunnel: w280 -> [w304 w337]
                tunnel: w277 -> [_ w334]
                frame False {
                  # "Magnetic Field plotting"
                  n125 = local read "Up/Down"() -> (w305:bool)
                  n126 = case shown="True" w305 {
                    frame True {
                      # "Down"
                      n127 = local read "I(B) 3"() -> (w315:cluster{dbl[], dbl[]}[])
                      n128 = local read "I(B) 3"() -> (w319:cluster{dbl[], dbl[]}[])
                      n129 = Index Array(array=w315, index=1) -> (element=w313:cluster{dbl[], dbl[]})
                      n130 = Unbundle(w313) -> (w312:dbl[], w311:dbl[])
                      n131 = Index Array(array=w319, index=i8 0 ("t")) -> (element=w316:cluster{dbl[], dbl[]})
                      n132 = local read "Actual Current (pA)"() -> (w308:dbl)
                      n133 = local read "Actual B Field (T)"() -> (w307:dbl)
                      n134 = Build Array (concatenate)(w312, w307) -> (w310:dbl[])
                      n135 = Build Array (concatenate)(w311, w308) -> (w309:dbl[])
                      n136 = Bundle(w310, w309) -> (w306:cluster{dbl[], dbl[]})  [unwired: 1 in]
                      n137 = Build Array(w316, w306) -> (w317:cluster{dbl[], dbl[]}[])
                      n138 = local write "I(B) 3"(w317) -> ()
                    }
                    frame False {
                      # "Up"
                      n139 = local read "I(B) 3"() -> (w331:cluster{dbl[], dbl[]}[])
                      n140 = local read "I(B) 3"() -> (w333:cluster{dbl[], dbl[]}[])
                      n141 = Index Array(array=w331, index=0) -> (element=w329:cluster{dbl[], dbl[]})
                      n142 = Unbundle(w329) -> (w328:dbl[], w327:dbl[])
                      n143 = Index Array(array=w333, index=i8 1 ("t")) -> (element=w321:cluster{dbl[], dbl[]})
                      n144 = local read "Actual B Field (T)"() -> (w323:dbl)
                      n145 = local read "Actual Current (pA)"() -> (w322:dbl)
                      n146 = Build Array (concatenate)(w328, w323) -> (w326:dbl[])
                      n147 = Build Array (concatenate)(w327, w322) -> (w325:dbl[])
                      n148 = Bundle(w326, w325) -> (w324:cluster{dbl[], dbl[]})  [unwired: 1 in]
                      n149 = Build Array(w324, w321) -> (w320:cluster{dbl[], dbl[]}[])
                      n150 = local write "I(B) 3"(w320) -> ()
                    }
                  }
                  n151 = Bundle(w302, w304) -> (→"P(B)":cluster{dbl[], dbl[]})  [unwired: 1 in]
                }
                frame True {
                  # "Temperature plotting"
                  n152 = Bundle(w336, w337) -> (→"P(T)":cluster{dbl[], dbl[]})  [unwired: 1 in]
                  n153 = Bundle(w336, w334) -> (→"I(T)":cluster{dbl[], dbl[]})  [unwired: 1 in]
                }
              }
            }
            frame "Save" {
              n154 = local read "Save"() -> (w339:dbl[][])
              n155 = local read "Counter"() -> (w355:i8)
              n156 = Build Array(w346, w345, w344, w343) -> (w342:dbl[][])
              n157 = Transpose 2D Array(2D array=w342) -> (transposed array=w341:dbl[][])
              n158 = local read "Reset"() -> (w352:bool)
              n159 = Greater?(x=w355, y=i8 0) -> (0:w351:bool)
              n160 = Build Array (concatenate)(w339, w341) -> (→"Save":dbl[][])
              n161 = And(x=w352, y=w351) -> (x .and. y?=w353:bool)
              n162 = case shown="True" w353 {
                tunnel: w344 -> [w364 w365]
                tunnel: [w364 w369] -> w350
                tunnel: w343 -> [w363 w366]
                tunnel: [w363 w369] -> w349
                tunnel: w345 -> [w362 w367]
                tunnel: [w362 w369] -> w348
                tunnel: w346 -> [w361 w368]
                tunnel: [w361 w369] -> w347
                frame False {
                }
                frame True {
                  n163 = stacked-sequence {
                    tunnel: [_ _ dbl[] []] -> w369
                    tunnel: w368 -> [_ _ w421]
                    tunnel: w367 -> [_ _ w425]
                    tunnel: w366 -> [_ w414 w419]
                    tunnel: w365 -> [_ w415 w420]
                    frame #0 {
                      n164 = local read "I(B) /Averaged/"() -> (w392:cluster{"B array":dbl[], dbl[]}[])
                      n165 = local read "I(B) 3"() -> (w399:cluster{dbl[], dbl[]}[])
                      n166 = Index Array(array=w399, index=0) -> (element=w398:cluster{dbl[], dbl[]})
                      n167 = Index Array(array=w399, index=1) -> (element=w400:cluster{dbl[], dbl[]})
                      n168 = local read "B array"() -> (w393:dbl[])
                      n169 = Index Array(array=w392, index=1) -> (element=w388:cluster{"B array":dbl[], dbl[]})
                      n170 = Unbundle(w398) -> (w396:dbl[], w397:dbl[])
                      n171 = Index Array(array=w392, index=0) -> (element=w389:cluster{"B array":dbl[], dbl[]})
                      n172 = Unbundle(w400) -> (w395:dbl[], w394:dbl[])
                      n173 = Unbundle(w388) -> ("B array"=w373:dbl[], w381:dbl[])
                      n174 = Unbundle(w389) -> ("B array"=w375:dbl[], w387:dbl[])
                      n175 = local read "Counter"() -> (w379:i8)
                      n176 = call <vilib>:"Interpolate 1D.vi"("xi"=w393, "X"=w395, "Y"=w394) -> ("yi"=w377:dbl[])  [unwired: 6 in, 2 out]
                      n177 = call <vilib>:"Interpolate 1D.vi"("xi"=w393, "X"=w396, "Y"=w397) -> ("yi"=w384:dbl[])  [unwired: 6 in, 2 out]
                      n178 = Decrement(x=w379) -> (x-1=w386:i8)
                      n179 = Decrement(x=w379) -> (x-1=w380:i8)
                      n180 = Multiply(x=w387, y=w386) -> (x*y=w385:dbl[])
                      n181 = Multiply(x=w381, y=w380) -> (x*y=w378:dbl[])
                      n182 = Add(x=w385, y=w384) -> (x+y=w383:dbl[])
                      n183 = Add(x=w377, y=w378) -> (x+y=w382:dbl[])
                      n184 = Divide(x=w383, y=w379) -> (x/y=w376:dbl[])
                      n185 = Divide(x=w382, y=w379) -> (x/y=w374:dbl[])
                      n186 = Bundle("B array"=w373, w374) -> (w371:cluster{"B array":dbl[], dbl[]})  [unwired: 1 in]
                      n187 = Bundle("B array"=w375, w376) -> (w372:cluster{"B array":dbl[], dbl[]})  [unwired: 1 in]
                      n188 = Build Array(w372, w371) -> (→"I(B) /Averaged/":cluster{"B array":dbl[], dbl[]}[])
                    }
                    frame #1 {
                      n189 = local read "B array"() -> (w407:dbl[])
                      n190 = local read "Counter"() -> (w413:i8)
                      n191 = local read "Averaged I(B)"() -> (w417:dbl[][])
                      n192 = local read "Up/Down"() -> (w416:bool)
                      n193 = Decrement(x=w413) -> (x-1=w403:i8)
                      n194 = call "Average_IB_curves.vi"("B array"=w407, "Up/Down"=w416, "Counter"=w403, "Array 3"=w415, "Averaged I(B)"=w417, "Array in"=w414) -> ("Averaged I(B) out"=w412:dbl[][])  [unwired: 5 in]
                      "Averaged I(B)" <- w412
                      n195 = Index Array(array=w412, index (col)=0 ("disabled index (col)")) -> (element=w409:dbl[])  [unwired: 1 in]
                      n196 = Index Array(array=w412, index (col)=1 ("disabled index (col)")) -> (element=w408:dbl[])  [unwired: 1 in]
                      n197 = Bundle("B array"=w407, "Averaged I(B) out"=w409) -> (w406:T6)  [unwired: 1 in]
                      n198 = Bundle("B array"=w407, "Averaged I(B) out"=w408) -> (w405:T6)  [unwired: 1 in]
                      n199 = Build Array(w406, w405) -> (→"I(B) /Averaged/ 2":T7)
                    }
                    frame #2 {
                      # "Save and Reset"
                      n200 = local read "P(uC/mm^2)"() -> (w418:dbl[])
                      n201 = Build Array(w425, w420, w419, w421, w418) -> (w422:dbl[][])
                      n202 = local read "output array"() -> (w424:dbl[][])
                      n203 = Build Array (concatenate)(w424, w422) -> (→"output array":dbl[][])
                      n204 = local write "Reset"(FALSE ("Save")) -> ()
                    }
                  }
                }
              }
            }
            frame "Return" {
            }
          }
        }
      }
      frame Error {
        # "Return true for any case which should stop the loop."
      }
    }
  }
  n205 = while {
    shift-right: [w456] -> w33
    shift-left: w9 -> [w457]
    shift-right: [w458] -> w40
    shift-left: w41 -> [w459]
    tunnel: w36 -> [w455]
    tunnel: w35 -> [w454]
    tunnel: w12 -> [w453]
    tunnel: [w447] -> _
    tunnel: w20 -> [w446]
    tunnel: w7 -> [w445]
    stop <- "stop" stop-if-true
    n206 = event shown="[5] \"Measure (Start/Pause)\": Value Change" {
      selector: _ -> [_ _ _ _ _ _ _ _ _ _ _ _ _]
      dyn-events: _ -> [_ _ _ _ _ _ _ _ _ _ _ _ _]
      timeout: 10 -> [_ _ _ _ _ _ _ _ _ _ _ _ _]
      tunnel: w459 -> [w469 w502 w512 w520 w531 w535 w556 _ w609 w616 w632 w642 w653]
      tunnel: [w468 w502 w512 w520 w531 w535 w556 _ w609 w616 w632 w642 w653] -> w458
      tunnel: w457 -> [w467 w501 w511 w521 w530 w539 w555 _ w610 w618 w636 w646 w655]
      tunnel: [w466 w501 w511 w521 w532 w539 w555 _ w610 w617 w635 w645 w654] -> w456
      tunnel: w455 -> [w465 _ _ _ _ _ _ _ _ _ _ _ _]
      tunnel: w454 -> [w464 _ _ _ _ _ _ _ _ _ _ _ _]
      tunnel: w453 -> [w463 _ _ _ _ _ _ _ _ _ _ _ _]
      tunnel: [w461 w500 w510 w519 w533 w536 w554 _ w608 w615 w633 w643 _] -> w447
      tunnel: w446 -> [w461 w500 w513 w519 w533 w536 w554 _ w608 w615 w633 w643 _]
      tunnel: w445 -> [_ _ _ _ _ _ _ _ _ w619 w634 w647 w652]
      event Timeout {
        n207 = event-data() -> ()  [unwired: 1 in, 3 out]
        n208 = case shown="True" "Measuring" {
          tunnel: w469 -> [w471 w490]
          tunnel: [w471 w489] -> w468
          tunnel: w467 -> [w470 _]
          tunnel: [w470 w488] -> w466
          tunnel: w465 -> [_ w481]
          tunnel: w464 -> [_ w480]
          tunnel: w463 -> [_ w475]
          frame False {
          }
          frame True {
            w478 = ":FETCh? " ("data")
            w482 = u32 1000 ("byte count")
            # "Generate the data here."
            n209 = case shown="No Error" w475 {
              selector: w475 -> [w492 w493]
              tunnel: [w492 w493] -> w474
              tunnel: [w491 _] -> w473
              frame No Error {
                n210 = Get Date/Time In Seconds() -> (seconds since 1Jan1904=w491:timestamp)
              }
              frame Error {
              }
            }
            n211 = VISA Write(VISA resource name=w481, write buffer=w478, error in (no error)=w474) -> (VISA resource name out=w487:refnum<visa-resource-name>, error out=w485:errorcluster)  [unwired: 1 out]
            n212 = VISA Write(VISA resource name=w480, write buffer=w478, error in (no error)=w485) -> (VISA resource name out=w486:refnum<visa-resource-name>, error out=w484:errorcluster)  [unwired: 1 out]
            n213 = VISA Read(VISA resource name=w487, byte count=w482, error in (no error)=w484) -> (read buffer=w476:string, error out=w483:errorcluster)  [unwired: 2 out]
            n214 = VISA Read(VISA resource name=w486, byte count=w482, error in (no error)=w483) -> (read buffer=w477:string, error out=w479:errorcluster)  [unwired: 2 out]
            n215 = Bundle("seconds since 1Jan1904"=w473, "read buffer"=w476, "read buffer"=w477) -> (w472:T5)  [unwired: 1 in]
            n216 = Enqueue Element(queue=w490, element=w472, error in (no error)=w479) -> (queue out=w489:refnum<queue>, error out=w488:errorcluster)  [unwired: 1 in, 1 out]
          }
        }
      }
      event "Max Field (T)": Value Change {
        n217 = event-data() -> ()  [unwired: 1 in, 6 out]
        n218 = Divide(x="Max Field (T)", y="dB (T)") -> (x/y=w497:dbl)
        n219 = Increment(x=w497) -> (x+1=w496:dbl)
        n220 = for {
          N: w496 -> [_]
          tunnel: "dB (T)" -> [w507]
          tunnel: [w504] -> w495 mode=indexing
          tunnel: "Min Field (T)" -> [w505]
          tunnel: [0.0] -> _ mode=indexing
          i -> [w509]
          n221 = Decrement(x=w509) -> (x-1=w508:i32)
          n222 = Multiply(x=w508, y=w507) -> (x*y=w506:dbl)
          n223 = Add(x=w506, y=w505) -> (x+y=w504:dbl)
        }
        "B array" <- w495
      }
      event "Sweep Rate (T/min)": Value Change {
        n224 = event-data() -> ("NewVal"=w517:dbl)  [unwired: 1 in, 5 out]
        n225 = Number To Fractional String(number=w517, precision (6)=i16 3) -> (F-format string=w515:string)  [unwired: 2 in]
        n226 = Concatenate Strings("T" ("format string"), w515) -> (w514:string)
        n227 = call "GPIB - BusCommand.vi"("Command"=w514, "Address"=w513) -> ("Address(thru)"=w510:T4)  [unwired: 1 out]
      }
      event "Field To Zero": Value Change {
        n228 = event-data() -> ()  [unwired: 1 in, 6 out]
        n229 = Two Button Dialog(message="Do you want to switch off the field?", 1:"No" ("F button name (\"Cancel\")"), 2:"Yes" ("T button name (\"OK\")")) -> (T button?=w525:bool)
        n230 = case shown="True" w525 {
          tunnel: w519 -> [_ w528]
          frame False {
          }
          frame True {
            n231 = local read "Sweep Rate (T/min)"() -> (w527:dbl)
            n232 = call "ips_switchHeaterOff.vi"("Instrument address"=w528, "Rate"=w527) -> ("B"=w526:dbl)
            n233 = local write "Actual Field (T)"(w526) -> ()
          }
        }
      }
      event "Go to Set": Value Change {
        n234 = event-data() -> ()  [unwired: 1 in, 6 out]
        n235 = call "Set_B.vi"("error in (no error)"=w530, "address string"="25", "Set Field (T)"="Set Field (T)") -> ("error out"=w532:errorcluster)  [unwired: 8 in]
      }
      event "Measure (Start/Pause)": Value Change {
        n236 = event-data() -> ("OldVal"=w537:bool, "NewVal"=w538:bool)  [unwired: 1 in, 4 out]
        n237 = local write "Measuring"(w538) -> ()
        n238 = case shown="True" w537 {
          frame False {
            n239 = local write "Temperature array"(dbl[] []) -> ()
          }
          frame True {
            # "Save data"
            n240 = case shown="True" "Temp/Magnetic Field" {
              tunnel: [w547 w548] -> w542
              frame False {
                n241 = local read "output array"() -> (w547:dbl[][])
              }
              frame True {
                n242 = local read "Magnetic Field (T)"() -> (w553:dbl[])
                n243 = local read "Measured Current (pA)"() -> (w552:dbl[])
                n244 = local read "Elapsed Time (s)"() -> (w550:dbl[])
                n245 = local read "Temperature array"() -> (w551:dbl[])
                n246 = local read "P(uC/mm^2)"() -> (w549:dbl[])
                n247 = Build Array(w551, w553, w552, w550, w549) -> (w548:dbl[][])
              }
            }
            n248 = local read "Measurement File"() -> (w544:path)
            n249 = call-poly <vilib>:"Write Delimited Spreadsheet.vi"("file path (dialog if empty)"=w544, "format (%.3f)"="%.5g", "2D data"=w542, "append to file? (F)"=TRUE, "transpose? (F)"=TRUE) -> ()  [unwired: 9 in, 2 out]
          }
        }
      }
      event "Measure Noise": Value Change {
        n250 = event-data() -> ("NewVal"=w557:bool)  [unwired: 1 in, 5 out]
        n251 = case shown="True" w557 {
          frame False {
          }
          frame True {
            n252 = local read "Gain (V/A)"() -> (w562:dbl)
            n253 = call "Noise_measurement.vi"("Gain (V/A)"=w562, "Cycles"="Cycles", "Lower Cut-Off"="Cut-Off Frequency", "minimum value"="minimum value", "Filter On"="Filter On", "maximum value"="maximum value", "physical channels"="physical channels", "rate"="Rate", "samples per channel"="Samples per channel") -> ("Current (pA) Filtered"=→"Current (pA) Filtered":waveform(dbl), "PSD (pA/Hz^1/2) Peaks Removed"=→"PSD (pA/Hz^1/2) Peaks Removed":cluster{"f0":dbl, "df":dbl, "magnitude":dbl[]}, "Current (pA)"=→"Current (pA)":dbl[], "PSD (pA/Hz^1/2)"=→"PSD (pA/Hz^1/2)":cluster{"f0":dbl, "df":dbl, "magnitude":dbl[]})  [unwired: 3 in]
          }
        }
      }
      event "Calibrate": Value Change {
        n254 = event-data() -> ()  [unwired: 1 in, 6 out]
        n255 = case shown="True" "Calibrate" {
          frame False {
          }
          frame True {
            w574 = dbl[] []
            n256 = while {
              shift-right: [w607] -> w572
              shift-left: dbl[][] [] -> [w606]
              shift-right: [w590] -> _
              shift-left: w574 -> [w602]
              shift-right: [w599] -> _
              shift-left: w574 -> [w601]
              shift-right: [w589] -> _
              shift-left: w574 -> [w600]
              shift-right: [w581] -> _
              shift-left: 0.0 ("Set Field out") -> [w580]
              stop <- w603 stop-if-true
              n257 = call "Calibtarion.vi"("Dwell Time (ms)"="Dwell Time (ms)", "V array in (V)"=w602, "I array in (A)"=w600, "Collected array in"=w606, "B array in (T)"=w601, "Set Field (T)"=w580, "dB"="dB") -> ("Best Linear Fit"=w591:dbl[], "appended array"=→"appended array":dbl[][], "slope"=→"B/V (T/V)":dbl, "V array out (V)"=w590:dbl[], "Boolean"=w605:bool, "I array out (A)"=w589:dbl[], "intercept 2"=→"I0 (A)":dbl, "Collected array out"=w607:dbl[][], "intercept"=→"B0 (T)":dbl, "B array Out"=w599:dbl[], "slope 2"=→"V/I (Ohm)":dbl, "Best Linear Fit 2"=w596:dbl[], "Set Field out"=w581:dbl)
              n258 = Bundle("I array out (A)"=w589, "V array out (V)"=w590) -> (w598:T8)  [unwired: 1 in]
              n259 = Bundle("I array out (A)"=w589, "Best Linear Fit"=w591) -> (w592:T9)  [unwired: 1 in]
              n260 = Bundle("V array out (V)"=w590, "B array Out"=w599) -> (w594:T10)  [unwired: 1 in]
              n261 = Bundle("V array out (V)"=w590, "Best Linear Fit 2"=w596) -> (w595:T11)  [unwired: 1 in]
              n262 = Or(x=w605, y="stop 2") -> (x .or. y?=w603:bool)
              n263 = Build Array(w598, w592) -> (→"V_I":T12)
              n264 = Build Array(w594, w595) -> (→"B_V":T13)
            }
            n265 = flat-sequence {
              tunnel: w572 -> [w578]
              frame #0 {
                n266 = Two Button Dialog(message="Do you want to save calibration file?") -> (T button?=w577:bool)  [unwired: 2 in]
                n267 = case shown="True" w577 {
                  tunnel: w578 -> [_ w579]
                  frame False {
                  }
                  frame True {
                    n268 = call-poly <vilib>:"Write Delimited Spreadsheet.vi"("2D data"=w579) -> ()  [unwired: 13 in, 2 out]
                  }
                }
              }
            }
          }
        }
      }
      event "New Measurement File": Value Change {
        n269 = event-data() -> ()  [unwired: 1 in, 6 out]
        n270 = Open/Create/Replace File(prompt="Please select measurement file\n", operation (0:open)=T3."replace or create with confirmation") -> (refnum out=w611:refnum<file>)  [unwired: 4 in, 2 out]
        n271 = local write "refnum out"(w611) -> ()
        n272 = Refnum to Path(1:w611) -> (0:w612:path)
        n273 = call "File_header_diag.vi"("Byte Stream File in"=w611) -> ()  [unwired: 11 in]
        n274 = local write "Measurement File"(w612) -> ()
      }
      event "Heater On/Off": Value Change {
        n275 = event-data() -> ()  [unwired: 1 in, 6 out]
        n276 = case shown="True" "Heater On/Off" {
          tunnel: w619 -> [w624 w630]
          tunnel: w618 -> [w622 w631]
          tunnel: [w621 w629] -> w617
          frame False {
            n277 = VISA Write(VISA resource name=w624, write buffer="RANGE,1,0", error in (no error)=w622) -> (error out=w621:errorcluster)  [unwired: 2 out]
          }
          frame True {
            n278 = Number To Decimal String(number="Heater Range") -> (decimal integer string=w627:string)  [unwired: 1 in]
            n279 = Concatenate Strings("RANGE,1," ("write buffer"), w627) -> (w625:string)
            n280 = VISA Write(VISA resource name=w630, write buffer=w625, error in (no error)=w631) -> (error out=w629:errorcluster)  [unwired: 2 out]
          }
        }
      }
      event "Set temperature (K)": Value Change {
        n281 = event-data() -> ()  [unwired: 1 in, 6 out]
        n282 = local read "Set temperature (K)"() -> (w637:dbl)
        n283 = Number To Fractional String(number=w637, precision (6)=i16 3) -> (F-format string=w640:string)  [unwired: 2 in]
        n284 = Concatenate Strings("SETP 1," ("write buffer"), w640) -> (w638:string)
        n285 = VISA Write(VISA resource name=w634, write buffer=w638, error in (no error)=w636) -> (error out=w635:errorcluster)  [unwired: 2 out]
      }
      event "Temp Ramping Rate (K/min)": Value Change {
        n286 = event-data() -> ()  [unwired: 1 in, 6 out]
        n287 = local read "Temp Ramping Rate (K/min)"() -> (w644:dbl)
        n288 = Number To Fractional String(number=w644, precision (6)=i16 1) -> (F-format string=w650:string)  [unwired: 2 in]
        n289 = Concatenate Strings("RAMP 1,1," ("string"), w650) -> (w649:string)
        n290 = VISA Write(VISA resource name=w647, write buffer=w649, error in (no error)=w646) -> (error out=w645:errorcluster)  [unwired: 2 out]
      }
      event "Heater Range": Value Change {
        n291 = event-data() -> ()  [unwired: 1 in, 6 out]
        n292 = local read "Heater On/Off"() -> (w656:bool)
        n293 = case shown="False" w656 {
          tunnel: w655 -> [w657 w662]
          tunnel: [w657 w661] -> w654
          tunnel: w652 -> [_ w660]
          frame False {
          }
          frame True {
            n294 = local read "Heater Range"() -> (w658:enum16{"Off", "Low", "Medium", "High"})
            n295 = Number To Decimal String(number=w658) -> (decimal integer string=w664:string)  [unwired: 1 in]
            n296 = Concatenate Strings("RANGE,1," ("write buffer"), w664) -> (w663:string)
            n297 = VISA Write(VISA resource name=w660, write buffer=w663, error in (no error)=w662) -> (error out=w661:errorcluster)  [unwired: 2 out]
          }
        }
      }
    }
    n298 = Reciprocal(x="Sampling rate (Hz)") -> (1/x=w451:dbl)
    n299 = Multiply(x=w451, y=1000.0) -> (x*y=w449:dbl)
    n300 = Wait Until Next ms Multiple(millisecond multiple=w449) -> ()  [unwired: 1 out]
  }
  n301 = local read "Lake Shore"() -> (w10:refnum<visa-resource-name>)
  n302 = local read "IV converter"() -> (w31:refnum<visa-resource-name>)
  n303 = local read "Magnetic Field"() -> (w30:refnum<visa-resource-name>)
  n304 = VISA Close(VISA resource name=w31, error in (no error)=w33) -> (error out=w34:errorcluster)
  n305 = VISA Close(VISA resource name=w30, error in (no error)=w34) -> (error out=w32:errorcluster)
  n306 = Release Queue(queue=w40, error in (no error)=w32) -> (error out=w26:errorcluster)  [unwired: 1 in, 2 out]
  n307 = Merge Errors(w26, w25) -> (w27:errorcluster)
  n308 = VISA Close(VISA resource name=w10, error in (no error)=w27) -> (error out=w24:errorcluster)
  n309 = local read "refnum out"() -> (w22:refnum<file>)
  n310 = Close File(refnum=w22, error in=w24) -> (error out=w23:errorcluster)  [unwired: 1 out]
  n311 = call <vilib>:"Simple Error Handler.vi"("error in (no error)"=w23) -> ()  [unwired: 4 in, 5 out]
